vi "All Firmware Data FGV.vi"(7 "All Firmware Data FGV States":T3, 8 "Error In":errorcluster, 9 "Firmwares":T2[][][](array[typedef]), 10 "Devices":T1[][](array[typedef]), 11 "Families":string[](array[string])) -> (0 "Error Out":errorcluster, 1 "Firmwares":T2[][][](array[typedef]), 2 "Devices":T1[][](array[typedef]), 3 "Families":string[](array[string]))   [LabVIEW 2020, in "LMH-LINX.lvlib"]
uses:
  LMH-LINX.lvlib
  Type Defs/All Firmware Data FGV States.ctl
  Type Defs/Device Firmware.ctl
  Type Defs/Device Data.ctl
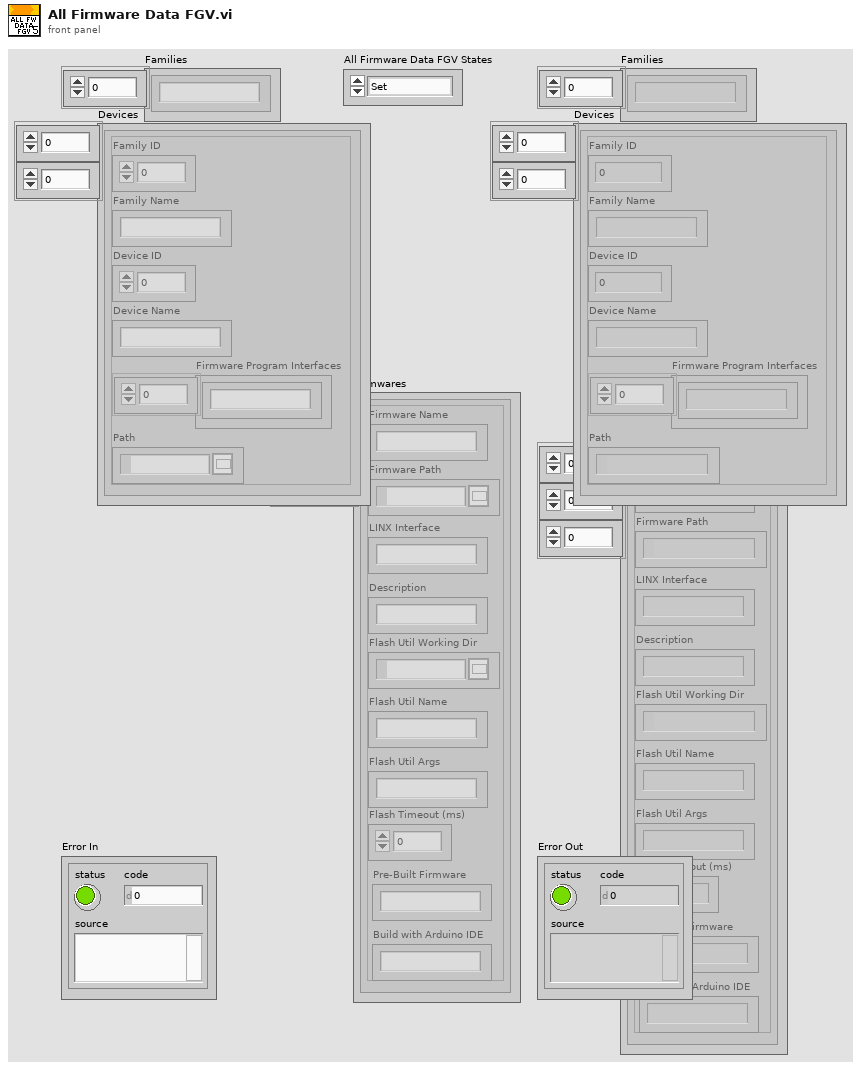
[diagram p1: front panel]
types:
  T1 = typedef "LMH-LINX.lvlib/Device Data.ctl" = cluster{"Family ID":i32, "Family Name":string, "Device ID":i32, "Device Name":string, "Firmware Program Interfaces":string[], "Path":path}
  T2 = typedef "LMH-LINX.lvlib/Device Firmware.ctl" = cluster{"Firmware Name":string, "Firmware Path":path, "Description":string, "LINX Interface":string, "Flash Util Working Dir":path, "Flash Util Name":string, "Flash Util Args":string, "Flash Timeout (ms)":i32, "Pre-Built Firmware":string, "Build with Arduino IDE":string}
  T3 = typedef "LMH-LINX.lvlib/All Firmware Data FGV States.ctl" = enum16{"Set", "Get"}
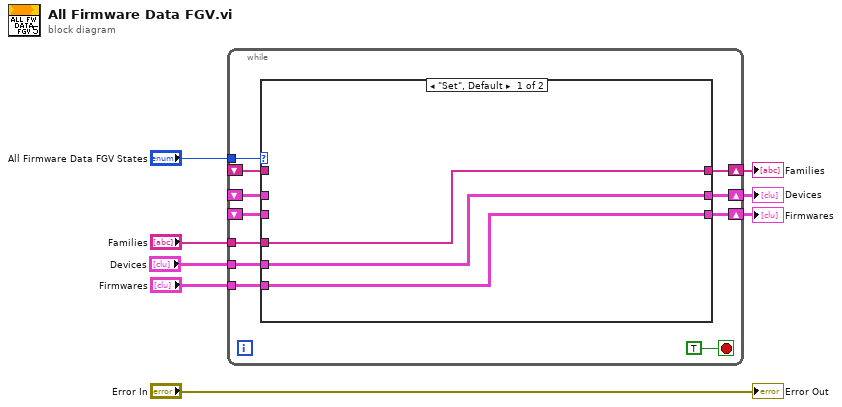
[diagram p0: block diagram]
diagram:
  n1 = while {
    tunnel: "All Firmware Data FGV States" -> [w18]
    shift-right: [w15] -> w5
    shift-left: _ -> [w16]
    shift-right: [w12] -> w4
    shift-left: _ -> [w17]
    tunnel: "Families" -> [w14]
    tunnel: "Firmwares" -> [w13]
    tunnel: "Devices" -> [w11]
    shift-right: [w10] -> w1
    shift-left: _ -> [w9]
    stop <- TRUE stop-if-true
    n2 = case shown="\"Set\", Default" w18 {
      tunnel: w17 -> [_ w24]
      tunnel: w16 -> [_ w25]
      tunnel: [w22 w25] -> w15
      tunnel: w14 -> [w22 _]
      tunnel: w13 -> [w21 _]
      tunnel: [w21 w24] -> w12
      tunnel: w11 -> [w20 _]
      tunnel: [w20 w23] -> w10
      tunnel: w9 -> [_ w23]
      frame "Set", Default {
      }
      frame "Get" {
      }
    }
  }
  "Families" <- w5
  "Firmwares" <- w4
  "Devices" <- w1
  "Error Out" <- "Error In"
